vi "Generatezlines_slower.vi"() -> ()   [LabVIEW 2018]
panel:
  in  "Offset Coordinates / nm":cluster{"X":dbl, "Y":dbl, "Z":dbl}={"X"=0.0, "Y"=0.0, "Z"=100.0} {"Z" min=0.0 max=1000.0 step=50.0}
  out "Output":dbl[][](graph)
  in  "Stop VI":bool
  in  "Amplitude/nm":dbl=100.0 min=0.0 max=1500.0 step=1.0
  in  "Sampling Rate / Hz":dbl=1000.0
  in  "Physical Channels":tag="PIEZO/ao0:2"
  # "Output Settings"
  # "Recommended sampling rate is 250Hz - each step in the stepping program will then be 1s of still followed by 0.2s of slew to next step level. Recommended Amplitude is 504nm and Offsets X: 0nm, \nY: 0nm, Z: 504 nm. You will need to navigate to your own physical channels where the piezo is attached. Usually the last 3 digits of this field read ' 0:2 ' when correctly configured.\n\nThis code is not really adjustable despite the fact it has controls - really only the offset and amplitude should be changed.\nThe sub VI's are not written flexibly so changing the number of samples will cause errors that may damage the piezo, so the number of samples is set at 12000.\n \nSlower sampling may cause timeout errors but these can be avoided by changing the timeout time in sub vi's.\nHigher sampling (>1000Hz) shouldn't be tried without checking the piezo manual for speed of voltage changes.  \n\nUsing the 'Stop' button to end the program is strongly recommended to avoid damaging the Piezo."
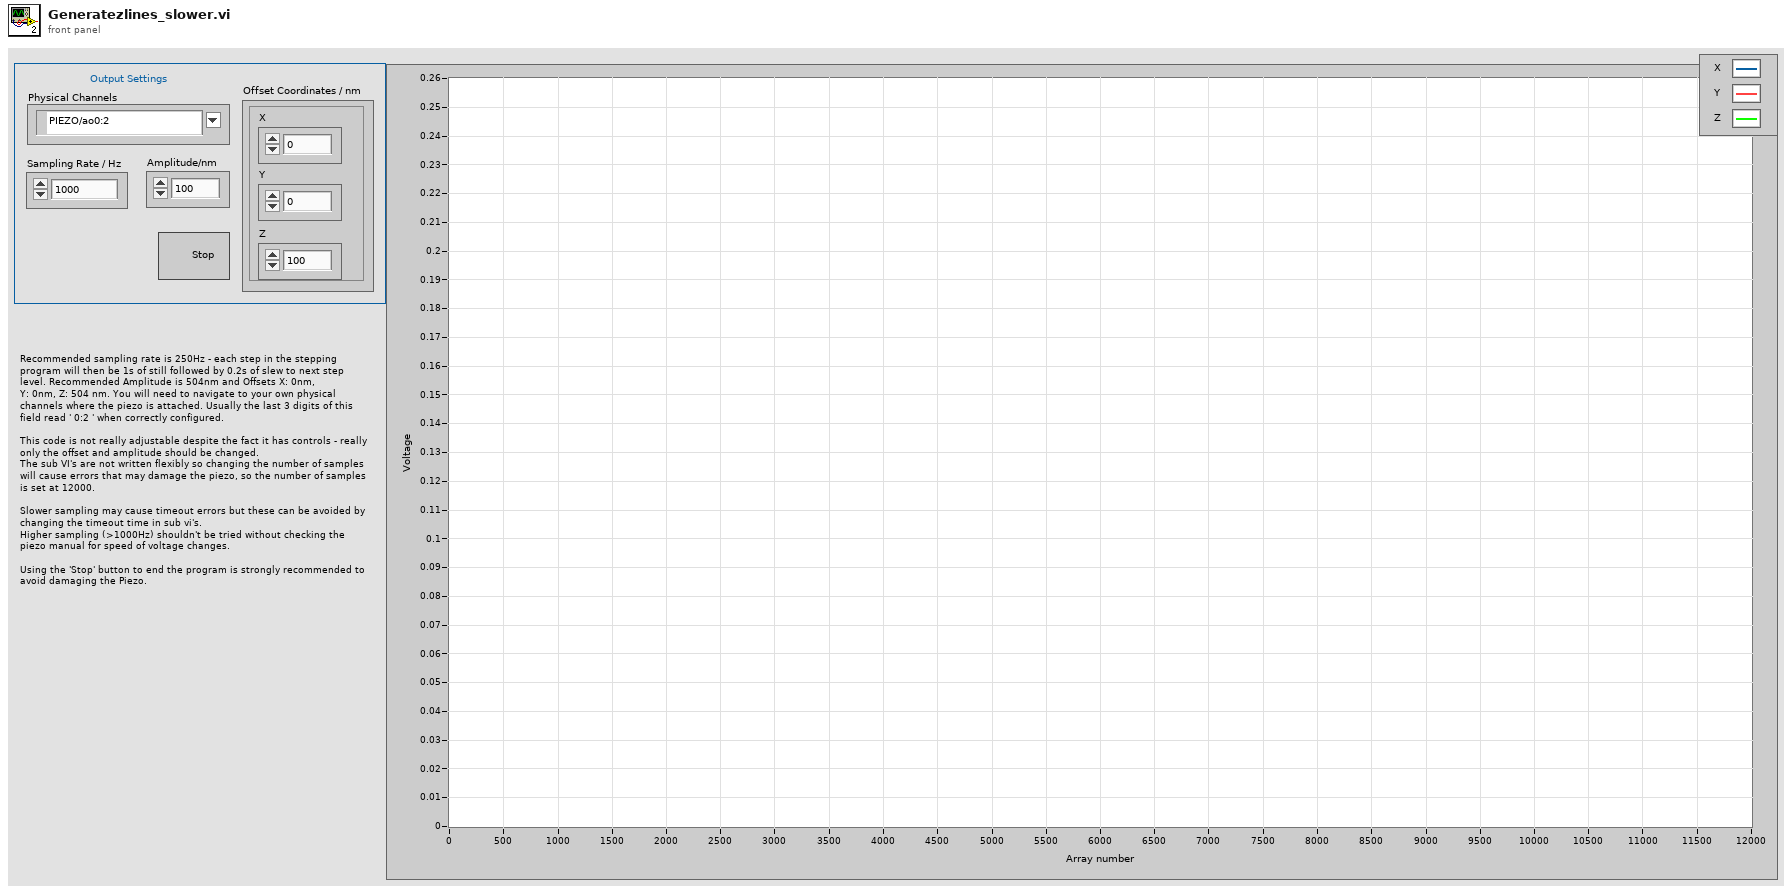
[diagram p1: front panel]
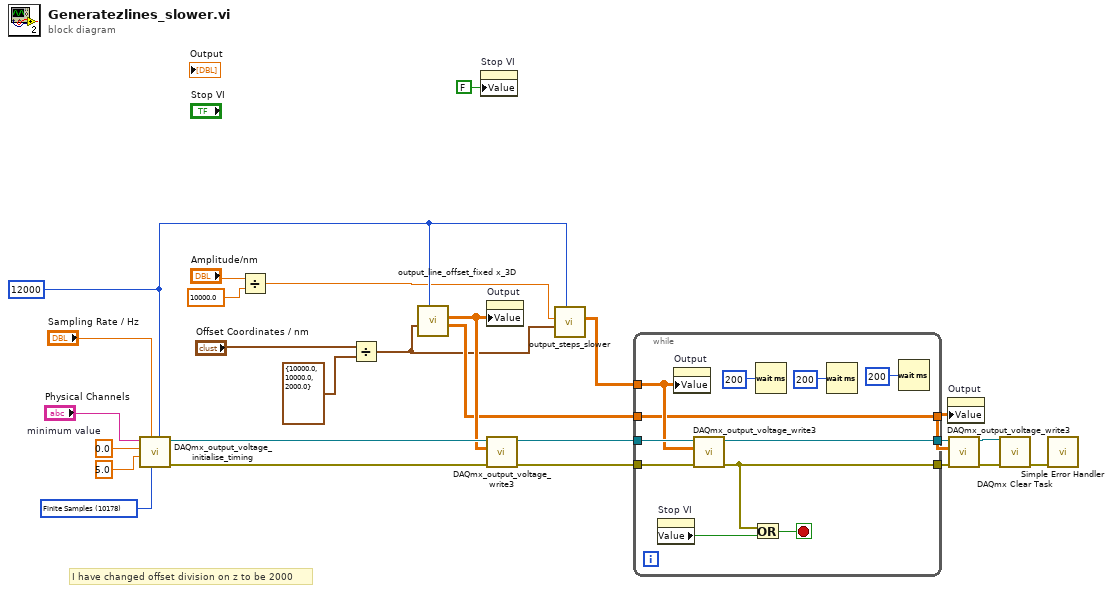
[diagram p0: block diagram]
diagram:
  w22 = 12000 ("Number of Samples")
  w3 = 10178 items=["Finite Samples"=10178, "Continuous Samples"=10123, "Hardware Timed Single Point"=12522] ("sample mode")
  w25 = 0.0  # minimum value
  # "I have changed offset division on z to be 2000"
  n1 = call "DAQmx_output_voltage_initialise_timing.vi"("samples per channel"=w22, "sample mode"=w3, "rate"="Sampling Rate / Hz", "maximum value"=5.0, "minimum value"=w25, "Physical Channels"="Physical Channels") -> ("error out"=w20:errorcluster, "task out"=w21:refnum<k21>)  [unwired: 4 in]
  n2 = Divide(x="Amplitude/nm", y=10000.0) -> (x/y=w1:dbl)
  n3 = Divide(x="Offset Coordinates / nm", y=cluster{"X":dbl, "Y":dbl, "Z":dbl} {"X"=10000.0, "Y"=10000.0, "Z"=2000.0}) -> (x/y=w2:cluster{"X":dbl, "Y":dbl, "Z":dbl})
  n4 = call "output_line_offset_fixed x_3D.vi"("# of samples"=w22, "Offset / V"=w2) -> ("Falling Slope"=w7:dbl[][], "Rising slope"=w13:dbl[][])  [unwired: 8 in]
  n5 = property on="Stop VI" class="Bool (strict)"("Value"=FALSE ("Stop VI")) -> ()  [unwired: 2 in, 2 out]
  n6 = property on="Output" class="WFGraph (strict)"("Value"=w13) -> ()  [unwired: 2 in, 2 out]
  n7 = call "DAQmx_output_voltage_write3.vi"("error in"=w20, "data"=w13, "task/channels in"=w21) -> ("error out"=w16:errorcluster, "task out"=w17:refnum<k21>)  [unwired: 7 in]
  n8 = call "output_steps_slower.vi"("# of Samples"=w22, "Offset / V"=w2, "Amplitude / V"=w1) -> ("Output"=w12:dbl[][])  [unwired: 8 in]
  n9 = while {
    tunnel: w17 -> [w37]
    tunnel: w16 -> [w36]
    tunnel: [w35] -> w15
    tunnel: [w33] -> w14
    tunnel: w12 -> [w34]
    tunnel: w7 -> [w30]
    tunnel: [w30] -> w6
    stop <- w31 stop-if-true
    n10 = property on="Stop VI" class="Bool (strict)"() -> ("Value"=w32:bool)  [unwired: 2 in, 2 out]
    n11 = property on="Output" class="WFGraph (strict)"("Value"=w34) -> ()  [unwired: 2 in, 2 out]
    n12 = call "DAQmx_output_voltage_write3.vi"("error in"=w36, "data"=w34, "task/channels in"=w37) -> ("error out"=w33:errorcluster, "task out"=w35:refnum<k21>)  [unwired: 7 in]
    n13 = Or(x=w33, y=w32) -> (x .or. y?=w31:bool)
    n14 = Wait (ms)(milliseconds to wait=u32 200) -> ()  [unwired: 1 out]
    n15 = Wait (ms)(milliseconds to wait=u32 200) -> ()  [unwired: 1 out]
    n16 = Wait (ms)(milliseconds to wait=u32 200) -> ()  [unwired: 1 out]
  }
  n17 = property on="Output" class="WFGraph (strict)"("Value"=w6) -> ()  [unwired: 2 in, 2 out]
  n18 = call "DAQmx_output_voltage_write3.vi"("error in"=w14, "data"=w6, "task/channels in"=w15) -> ("error out"=w9:errorcluster, "task out"=w8:refnum<k21>)  [unwired: 7 in]
  n19 = call <vilib>:"DAQmx Clear Task.vi"("task in"=w8, "error in"=w9) -> ("error out"=w10:errorcluster)  [unwired: 13 in]
  n20 = call <vilib>:"Simple Error Handler.vi"("error in (no error)"=w10) -> ()  [unwired: 4 in, 5 out]
